vi "memory leaks.vi"() -> ()   [LabVIEW 2021]
uses:
  Source/Open Xml.lvlib
panel:
  out "Cells":string[][](array[string])
  out "Value String":string
  out "error out":errorcluster
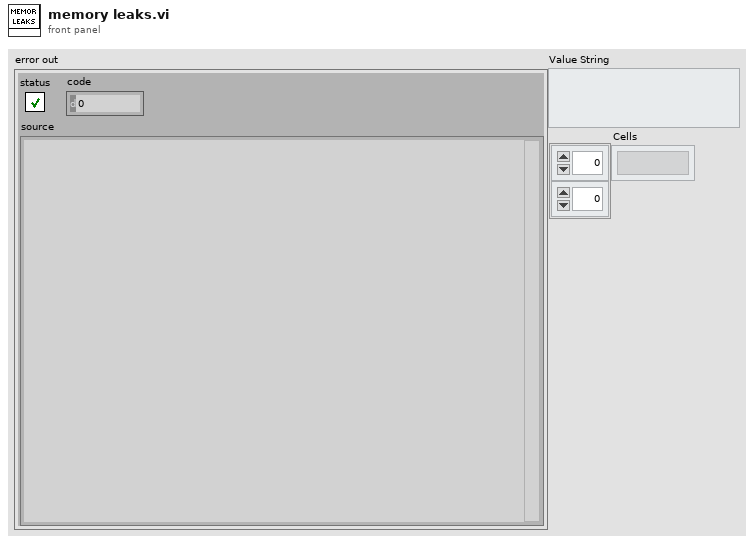
[diagram p1: front panel]
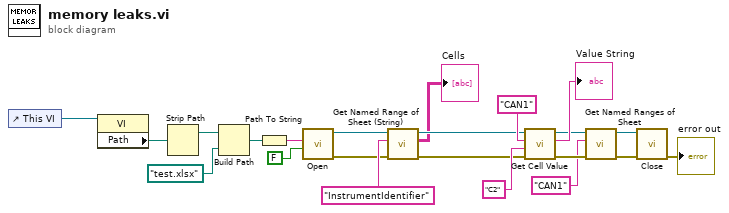
[diagram p0: block diagram]
diagram:
  n1 = control-ref of="This VI"() -> (w22:refnum<vi>)
  n2 = property class="VI"(reference=w22) -> ("Path"=w21:path)  [unwired: 1 in, 2 out]
  n3 = Strip Path(path=w21) -> (stripped path=w20:path)  [unwired: 1 out]
  n4 = Build Path(base path=w20, name or relative path=path "test.xlsx") -> (appended path=w18:path)
  n5 = Path To String(path=w18) -> (string=w17:string)
  n6 = call "Open.vi"("isEditable"=FALSE, "Path"=w17) -> ("error out"=w6:errorcluster, "SpreadsheetDocument"=w5:refnum<k24>)  [unwired: 8 in]
  n7 = call "Get Named Range of Sheet (String).vi"("error in"=w6, "Named Range Identifier"="InstrumentIdentifier", "SpreadsheetDocument"=w5) -> ("error out"=w10:errorcluster, "Cells"=→"Cells":string[][], "SpreadsheetDocument out"=w9:refnum<k24>)  [unwired: 6 in]
  n8 = call "Get Cell Value.vi"("error in"=w10, 9:"C2" ("Cell Address"), "Cell Address"="CAN1" ("Sheet Name"), "SpreadsheetDocument"=w9) -> ("error out"=w13:errorcluster, "Value String"=→"Value String":string, "SpreadsheetDocument out"=w3:refnum<k24>)  [unwired: 2 in, 3 out]
  n9 = call "Get Named Ranges of Sheet.vi"("error in"=w13, "Sheet Name"="CAN1", "SpreadsheetDocument"=w3) -> ("error out"=w4:errorcluster, "SpreadsheetDocument out"=w2:refnum<k24>)  [unwired: 5 in, 2 out]
  n10 = call "Close.vi"("error in"=w4, "SpreadsheetDocument"=w2) -> ("error out"=→"error out":errorcluster)  [unwired: 9 in]
